vi "MGCC_StaEst_initial_4.vi"() -> ()   [LabVIEW 2016]
uses:
  <vilib>/imath/engines/lvmath2/RunTimeEngine/RunTimeType/NIMS_RunTimeType_From StrictType (excl LVString).vi
  <instcachedir>/0/NIMS_RunTimeType_From StrictType (excl LVString)_BBF44FB49F834B71AF7A14CCEDF8BECD.lvgen/NIMS_RunTimeType_From StrictType (excl LVString)_BBF44FB49F834B71AF7A14CCEDF8BECD_010.vi
  <vilib>/imath/engines/lvmath2/RunTimeEngine/Struct/NIMS_StructSetField.vi
  <instcachedir>/0/NIMS_RunTimeType_From StrictType (excl LVString)_BBF44FB49F834B71AF7A14CCEDF8BECD.lvgen/NIMS_RunTimeType_From StrictType (excl LVString)_BBF44FB49F834B71AF7A14CCEDF8BECD_032.vi
  <instcachedir>/0/NIMS_RunTimeType_From StrictType (excl LVString)_BBF44FB49F834B71AF7A14CCEDF8BECD.lvgen/NIMS_RunTimeType_From StrictType (excl LVString)_BBF44FB49F834B71AF7A14CCEDF8BECD_031.vi
  <instcachedir>/0/NIMS_RunTimeType_From StrictType (excl LVString)_BBF44FB49F834B71AF7A14CCEDF8BECD.lvgen/NIMS_RunTimeType_From StrictType (excl LVString)_BBF44FB49F834B71AF7A14CCEDF8BECD_009.vi
  <instcachedir>/0/NIMS_RunTimeType_From StrictType (excl LVString)_BBF44FB49F834B71AF7A14CCEDF8BECD.lvgen/NIMS_RunTimeType_From StrictType (excl LVString)_BBF44FB49F834B71AF7A14CCEDF8BECD_000.vi
  <vilib>/imath/engines/lvmath2/RunTimeEngine/Struct/NIMS_StructGetField.vi
  <vilib>/imath/engines/lvmath2/RunTimeEngine/RunTimeType/NIMS_RunTimeType_To Numeric.vi
  <instcachedir>/0/NIMS_RunTimeType_To Numeric_19D51BCABB82435A94073491761E42EE.lvgen/NIMS_RunTimeType_To Numeric_19D51BCABB82435A94073491761E42EE_003.vi
  <vilib>/imath/engines/lvmath2/RunTimeEngine/ArithmeticOperatorToken/NIMS_ArithmeticOperator_times.vi
  <instcachedir>/0/NIMS_ArithmeticOperator_times_953B34F74CAC448FB707D816A29CC5F0.lvgen/NIMS_ArithmeticOperator_times_953B34F74CAC448FB707D816A29CC5F0_007.vi
  <vilib>/imathl/engines/lvmath/Functions/Error Handling/Create Error.vi
  <instcachedir>/0/NIMS_RunTimeType_To Numeric_19D51BCABB82435A94073491761E42EE.lvgen/NIMS_RunTimeType_To Numeric_19D51BCABB82435A94073491761E42EE_009.vi
  <vilib>/imath/engines/lvmath2/RunTimeEngine/BuiltInFunctions/reshapemx/NIMS_[GV]_reshapemx.vi
  <instcachedir>/0/NIMS_[GV]_reshapemx_314E456D64644EB191D4916921E89AA6.lvgen/NIMS_[GV]_reshapemx_314E456D64644EB191D4916921E89AA6_000.vi
  <instcachedir>/0/NIMS_RunTimeType_To Numeric_19D51BCABB82435A94073491761E42EE.lvgen/NIMS_RunTimeType_To Numeric_19D51BCABB82435A94073491761E42EE_004.vi
  <vilib>/imath/engines/lvmath2/RunTimeSupport/NIMS_Error if Not Equal.vi
  <instcachedir>/0/NIMS_Error if Not Equal_43252A79AD05436189442EC0C5E5AB8A.lvgen/NIMS_Error if Not Equal_43252A79AD05436189442EC0C5E5AB8A_001.vi
  <vilib>/imath/engines/lvmath2/RunTimeEngine/IndexRead/NIMS M(V).vi
  <instcachedir>/0/NIMS M(V)_948FAC22C1C943948B75DA6190348614.lvgen/NIMS M(V)_948FAC22C1C943948B75DA6190348614_005.vi
  <vilib>/imath/engines/lvmath2/RunTimeEngine/MatrixToken/NIMS_MatrixToken_M_M.vi
  <instcachedir>/0/NIMS_MatrixToken_M_M_DF273B0CC20F424BBF1EDA9F4E71C841.lvgen/NIMS_MatrixToken_M_M_DF273B0CC20F424BBF1EDA9F4E71C841_004.vi
  <vilib>/imath/engines/lvmath2/RunTimeEngine/ErrorHandling/NIMS_Create Error From Enums.vi
  <vilib>/imath/engines/lvmath2/RunTimeEngine/IndexRead/NIMS M($,S).vi
  <instcachedir>/0/NIMS M($,S)_3E5749BBB62E49528D4765A77F1F6D98.lvgen/NIMS M($,S)_3E5749BBB62E49528D4765A77F1F6D98_000.vi
  <vilib>/imath/engines/lvmath2/RunTimeEngine/NodeEndStatement/NIMS_NodeEndStatement_Output.vi
  <instcachedir>/0/NIMS_NodeEndStatement_Output_53EC0D466D134D7ABD903AC30B43404B.lvgen/NIMS_NodeEndStatement_Output_53EC0D466D134D7ABD903AC30B43404B_005.vi
  <instcachedir>/0/NIMS_NodeEndStatement_Output_53EC0D466D134D7ABD903AC30B43404B.lvgen/NIMS_NodeEndStatement_Output_53EC0D466D134D7ABD903AC30B43404B_025.vi
  <vilib>/imath/engines/lvmath2/RunTimeEngine/ErrorHandling/NIMS_Finalize Error.vi
panel:
  out "PN":dbl[][](array[numeric])
  out "error out 2":errorcluster
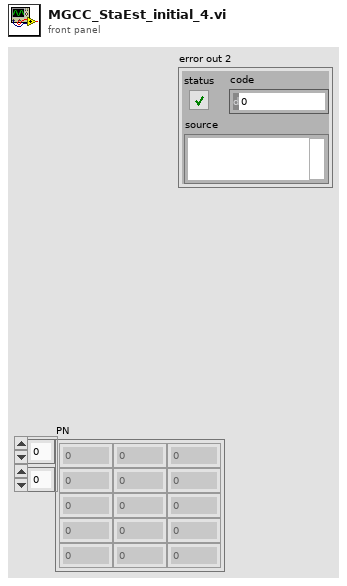
[diagram p1: front panel]
types:
  T1 = cluster{"PN":dbl[][], "QN":dbl[][], "VN":dbl[][]}
  T2 = cluster{"Node":dbl, "Line":dbl, "StateVar":i32, "Zeroinj":i32}
  T3 = cluster{"VOL":cdb[][], "PN":dbl[][], "QN":dbl[][], "IN":dbl[][], "Ve":dbl[][], "Vf":dbl[][], "VN":dbl[][], "AN":dbl[][]}
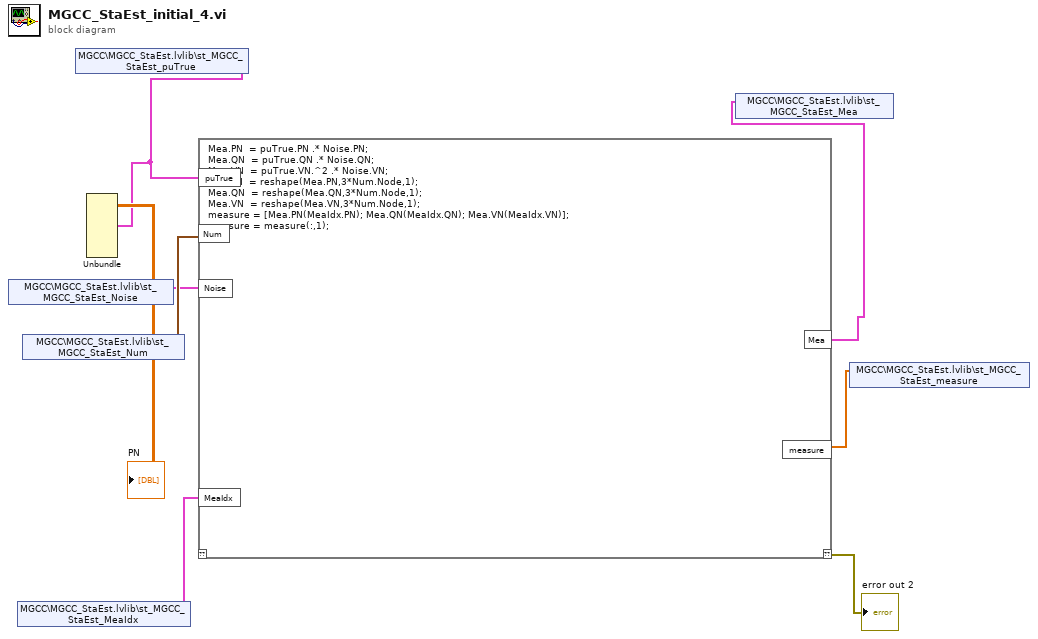
[diagram p0: block diagram]
diagram:
  n1 = shared-variable "MGCC\\MGCC_StaEst.lvlib\\st_MGCC_StaEst_Noise"() -> (w3:T1)  [unwired: 1 in, 1 out]
  n2 = shared-variable "MGCC\\MGCC_StaEst.lvlib\\st_MGCC_StaEst_MeaIdx"() -> (w4:cluster{"PN":dbl[], "QN":dbl[], "VN":dbl[]})  [unwired: 1 in, 1 out]
  n3 = shared-variable "MGCC\\MGCC_StaEst.lvlib\\st_MGCC_StaEst_Num"() -> (w5:T2)  [unwired: 1 in, 1 out]
  n4 = shared-variable "MGCC\\MGCC_StaEst.lvlib\\st_MGCC_StaEst_puTrue"() -> (w6:T3)  [unwired: 1 in, 1 out]
  n5 = Unbundle(w6) -> ("PN"=→"PN":dbl[][])  [unwired: 7 out]
  n6 = mathscript code="Mea.PN  = puTrue.PN .* Noise.PN; \nMea.QN  = puTrue.QN .* Noise.QN;\nMea.VN  = puTrue.VN.^2 .* Noise.VN;\nMea.PN  = reshape(Mea.PN,3*Num.Node,1);\nMea.QN  = reshape(Mea.QN,3*Num.Node,1);\nMea.VN  = reshape(Mea.VN,3*Num.Node,1);\nmeasure = [Mea.PN(MeaIdx.PN); Mea.QN(MeaIdx.QN); Mea.VN(MeaIdx.VN)];\nmeasure = measure(:,1);"("puTrue"=w6, "Noise"=w3, "Num"=w5, "MeaIdx"=w4) -> ("??"=→"error out 2":errorcluster, "Mea"=w2:T1, "measure"=w1:dbl[])  [unwired: 1 in]
  n7 = shared-variable "MGCC\\MGCC_StaEst.lvlib\\st_MGCC_StaEst_Mea"(w2) -> ()  [unwired: 1 in, 1 out]
  n8 = shared-variable "MGCC\\MGCC_StaEst.lvlib\\st_MGCC_StaEst_measure"(w1) -> ()  [unwired: 1 in, 1 out]
